vi "Send Publish Signal Message.vi"(8 "error in":errorcluster, 9 "Variant":variant, 10 "Signal Name":string, 11 "Actor Class":T1) -> (0 "error out":errorcluster)   [LabVIEW 2019]
uses:
  Actor Private Data.ctl
  <vilib>/LabVIEW Open Source Project/MQTT Client/Client class/Client.lvclass
  Actor Private Events -- cluster.ctl
  Payload -- cluster.ctl
  6952da43-da3b-427e-8764-0837e8a730c5.vi
  <vilib>/JDP Science/JSONtext/Variant to JSON Text.vi
  <vilib>/JDP Science/JSONtext/LVClass Serializer/JSONtext LVClass Serializer.lvclass
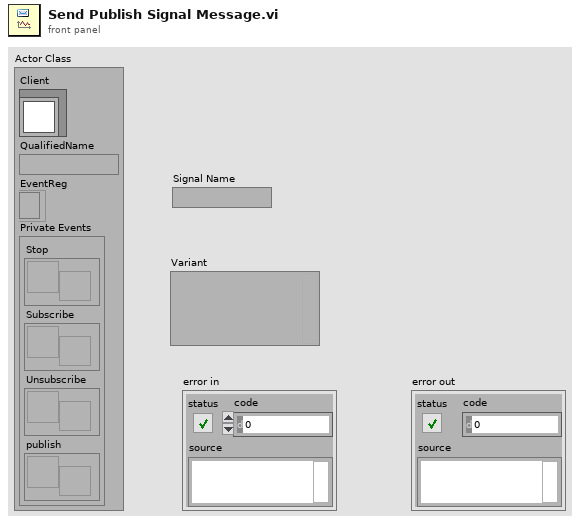
[diagram p1: front panel]
types:
  T1 = typedef "Actor Private Data.ctl" = cluster{"Client":refnum<class "Client.lvclass">, "QualifiedName":string, "EventReg":refnum<event-registration>, "Private Events":T2}
  T2 = typedef "Actor Private Events -- cluster.ctl" = cluster{"Stop":refnum<user-event>, "Subscribe":refnum<user-event>, "Unsubscribe":refnum<user-event>, "publish":refnum<user-event>}
  T3 = typedef "Payload -- cluster.ctl" = cluster{"topic":string, "Payload":u8[]}
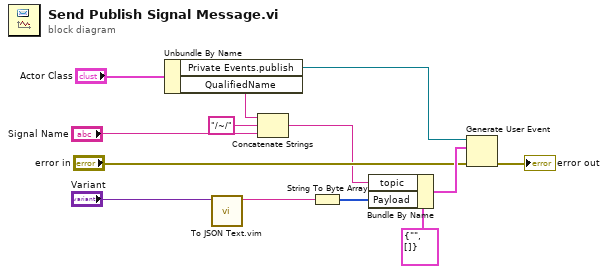
[diagram p0: block diagram]
diagram:
  n1 = Unbundle By Name("Actor Class") -> ("Private Events.publish"=w11:refnum<user-event>, "QualifiedName"=w6:string)
  n2 = call "To JSON Text.vim"("Anything"="Variant") -> ("<JSON>"=w1:string)  [unwired: 9 in, 1 out]
  n3 = Concatenate Strings(w6, "/~/" ("string"), "Signal Name") -> (w4:string)
  n4 = String To Byte Array(string=w1) -> (unsigned byte array=w3:u8[])
  n5 = Bundle By Name(cluster=T3 {"topic"="", "Payload"=[]} ("publish"), "topic"=w4, "Payload"=w3) -> (w10:T3)
  n6 = Generate User Event(user event=w11, event data cluster=w10, error in="error in") -> (error out=→"error out":errorcluster)  [unwired: 1 in, 1 out]
